vi "MD420_ACT_TargetValue.vi"() -> ()   [LabVIEW 2022 SP3, in "MD420.lvclass"]
uses:
  MD420.lvclass
  MD420.lvclass/MD420.ctl
  SI_modules/SI657/SI657.lvclass
  SI_modules/SI656/SI656.lvclass
  SI_modules/SI101/SI101_AverageReactorCoolantTemperature.lvclass
panel:
  in  "Redundacy Inputs":T1
  out "error IO":errorcluster
  in  "error in (no error)":errorcluster
  out "SI101_AverageReactorCoolantTemperature.lvclass out":refnum<class "SI101_AverageReactorCoolantTemperature.lvclass">
  out "SI657.lvclass out":refnum<class "SI657.lvclass">
  out "SI656 out":refnum<class "SI656.lvclass">
  in  "Loop Meas":T2
  in  "From Turbine SI656":T3
  in  "From Turbine SI657":T4
  in  "SI101_AverageReactorCoolantTemperature.lvclass":refnum<class "SI101_AverageReactorCoolantTemperature.lvclass">
  in  "SI656.lvclass":refnum<class "SI656.lvclass">
  in  "SI657.lvclass":refnum<class "SI657.lvclass">
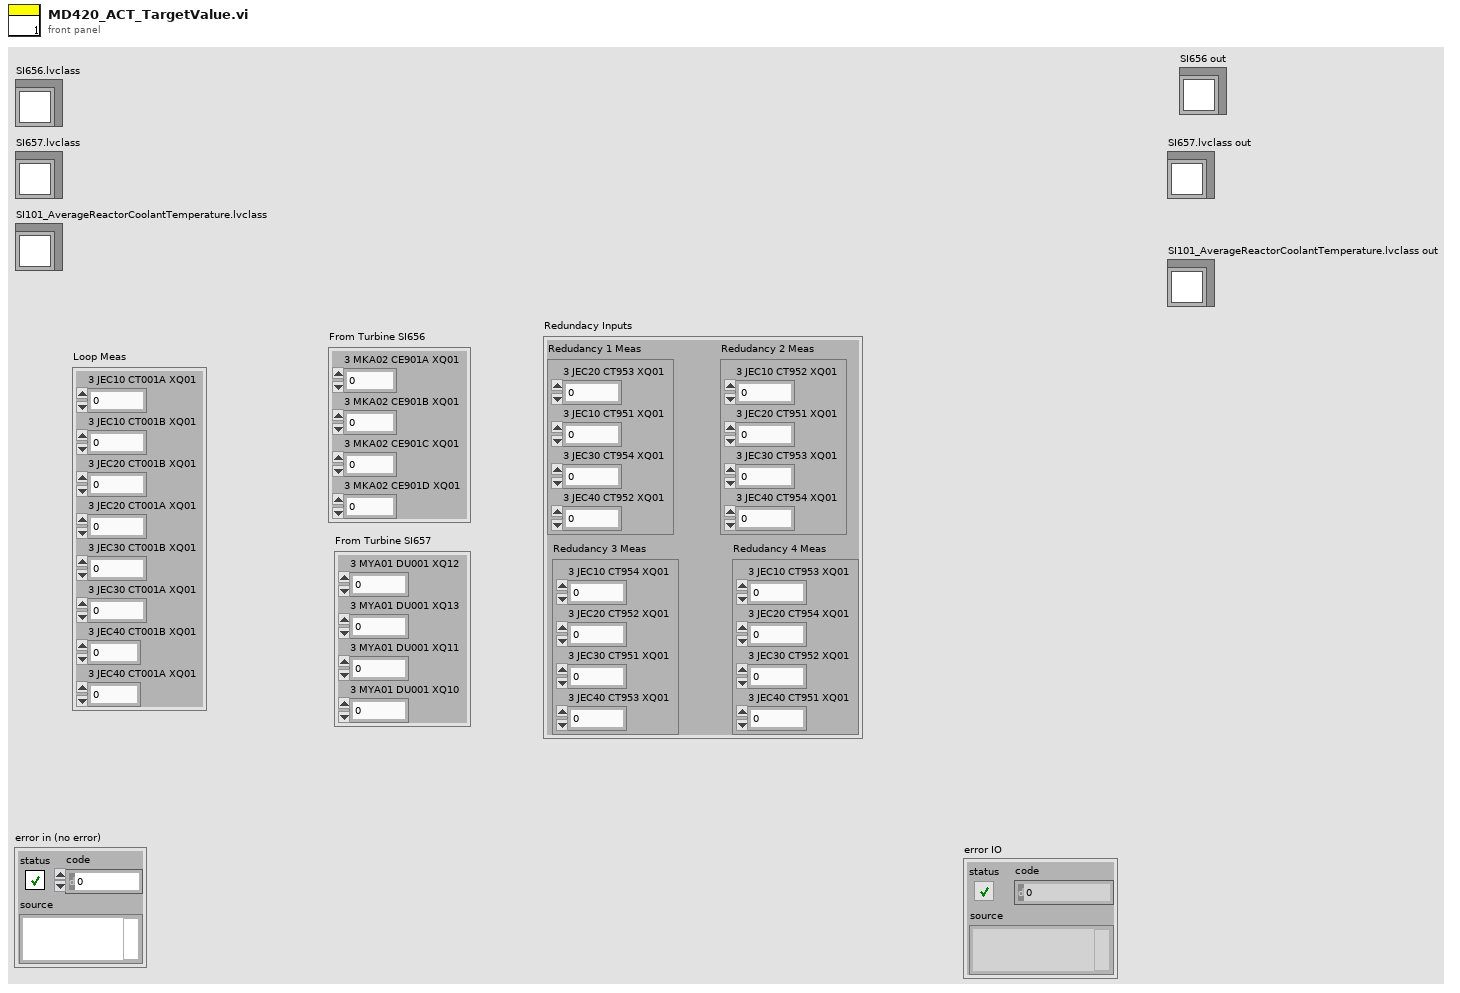
[diagram p1: front panel]
types:
  T1 = cluster{"Redudancy 1 Meas":cluster{"3 JEC20 CT953 XQ01":dbl, "3 JEC10 CT951 XQ01":dbl, "3 JEC30 CT954 XQ01":dbl, "3 JEC40 CT952 XQ01":dbl}, "Redudancy 2 Meas":cluster{"3 JEC10 CT952 XQ01":dbl, "3 JEC20 CT951 XQ01":dbl, "3 JEC30 CT953 XQ01":dbl, "3 JEC40 CT954 XQ01":dbl}, "Redudancy 3 Meas":cluster{"3 JEC10 CT954 XQ01":dbl, "3 JEC20 CT952 XQ01":dbl, "3 JEC30 CT951 XQ01":dbl, "3 JEC40 CT953 XQ01":dbl}, "Redudancy 4 Meas":cluster{"3 JEC10 CT953 XQ01":dbl, "3 JEC20 CT954 XQ01":dbl, "3 JEC30 CT952 XQ01":dbl, "3 JEC40 CT951 XQ01":dbl}}
  T2 = cluster{"3 JEC10 CT001A XQ01":dbl, "3 JEC10 CT001B XQ01":dbl, "3 JEC20 CT001B XQ01":dbl, "3 JEC20 CT001A XQ01":dbl, "3 JEC30 CT001B XQ01":dbl, "3 JEC30 CT001A XQ01":dbl, "3 JEC40 CT001B XQ01":dbl, "3 JEC40 CT001A XQ01":dbl}
  T3 = cluster{"3 MKA02 CE901A XQ01":dbl, "3 MKA02 CE901B XQ01":dbl, "3 MKA02 CE901C XQ01":dbl, "3 MKA02 CE901D XQ01":dbl}
  T4 = cluster{"3 MYA01 DU001 XQ12":dbl, "3 MYA01 DU001 XQ13":dbl, "3 MYA01 DU001 XQ11":dbl, "3 MYA01 DU001 XQ10":dbl}
  T5 = cluster{"3 JEC20 CT953 XQ01":dbl, "3 JEC10 CT951 XQ01":dbl, "3 JEC30 CT954 XQ01":dbl, "3 JEC40 CT952 XQ01":dbl}
  T6 = cluster{"3 JEC10 CT952 XQ01":dbl, "3 JEC20 CT951 XQ01":dbl, "3 JEC30 CT953 XQ01":dbl, "3 JEC40 CT954 XQ01":dbl}
  T7 = cluster{"3 JEC10 CT954 XQ01":dbl, "3 JEC20 CT952 XQ01":dbl, "3 JEC30 CT951 XQ01":dbl, "3 JEC40 CT953 XQ01":dbl}
  T8 = cluster{"3 JEC10 CT953 XQ01":dbl, "3 JEC20 CT954 XQ01":dbl, "3 JEC30 CT952 XQ01":dbl, "3 JEC40 CT951 XQ01":dbl}
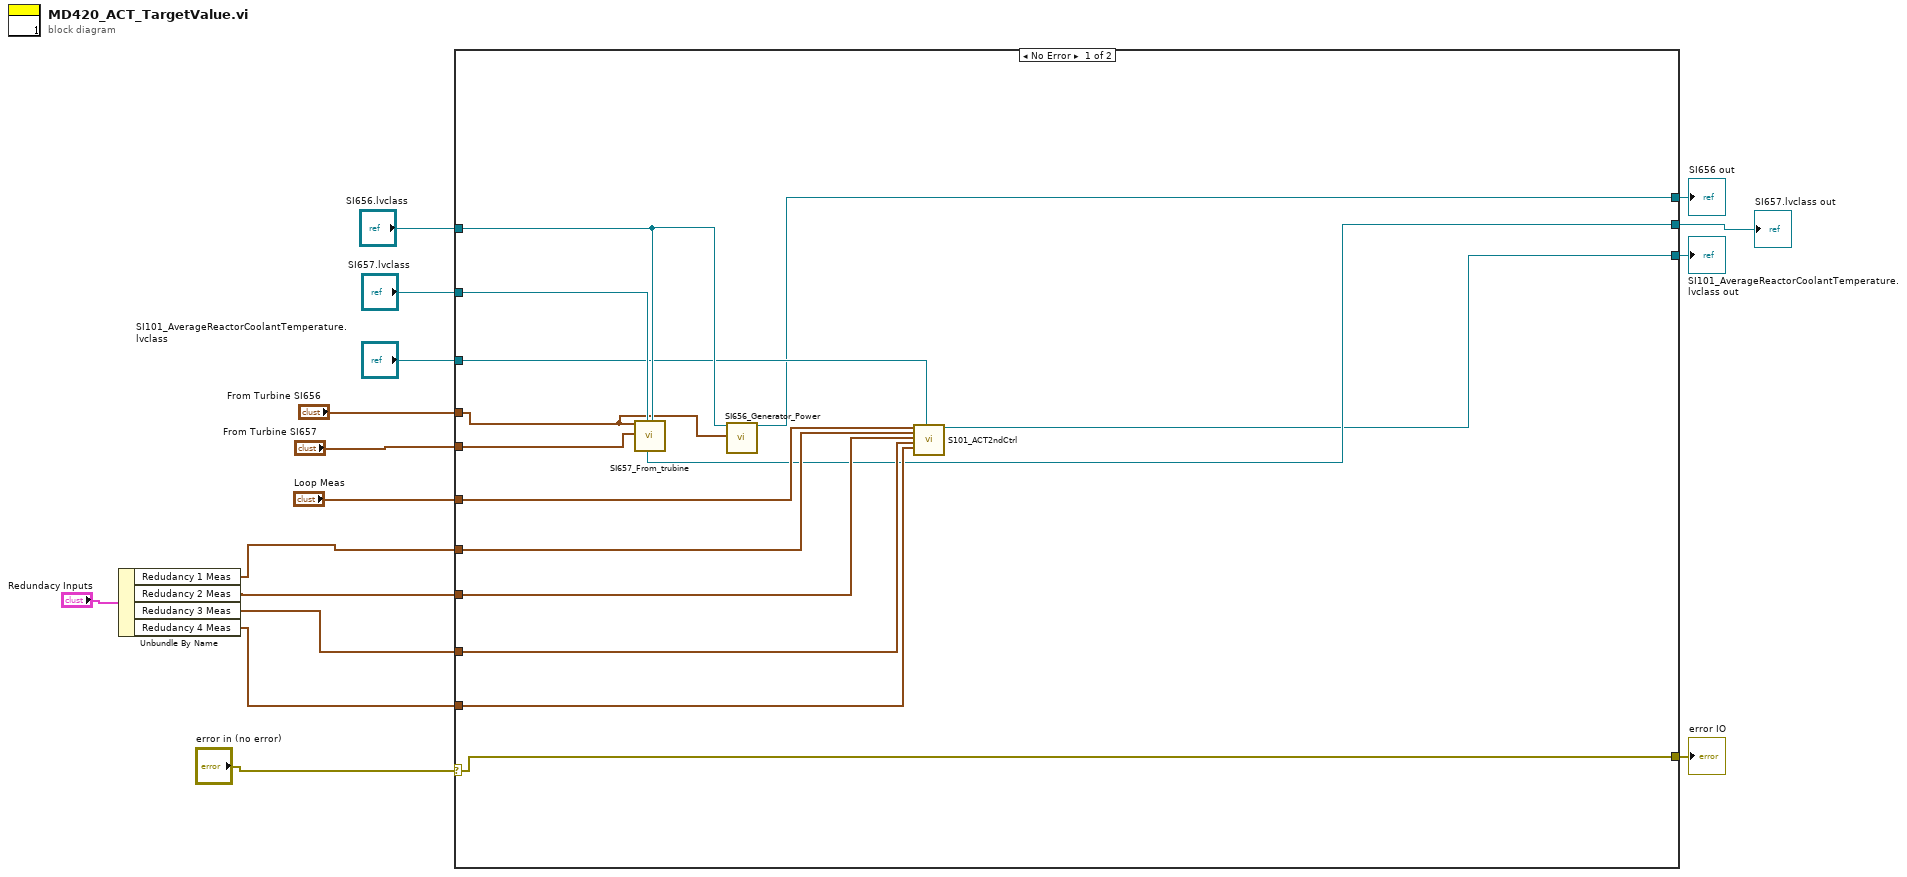
[diagram p0: block diagram]
diagram:
  n1 = Unbundle By Name("Redundacy Inputs") -> ("Redudancy 1 Meas"=w4:T5, "Redudancy 2 Meas"=w3:T6, "Redudancy 3 Meas"=w2:T7, "Redudancy 4 Meas"=w1:T8)
  n2 = case shown="No Error" "error in (no error)" {
    selector: "error in (no error)" -> [w17 w31]
    tunnel: "SI657.lvclass" -> [w30 _]
    tunnel: "SI656.lvclass" -> [w28 _]
    tunnel: "SI101_AverageReactorCoolantTemperature.lvclass" -> [w26 _]
    tunnel: "From Turbine SI656" -> [w27 _]
    tunnel: "From Turbine SI657" -> [w29 _]
    tunnel: "Loop Meas" -> [w25 _]
    tunnel: w4 -> [w24 _]
    tunnel: w3 -> [w23 _]
    tunnel: w2 -> [w22 _]
    tunnel: w1 -> [w21 _]
    tunnel: [w20 _] -> w9
    tunnel: [w19 _] -> w10
    tunnel: [w18 _] -> w8
    tunnel: [w17 w31] -> w6
    frame No Error {
      n3 = call "SI657_From_trubine.vi"("From Turbine SI656"=w27, "From Turbine SI657"=w29, "SI657.lvclass"=w30, "SI656.lvclass"=w28) -> ("SI657.lvclass out"=w20:refnum<class "SI657.lvclass">)  [unwired: 8 in, 7 out]
      n4 = call "SI656_Generator_Power.vi"("SI656 in"=w28, "From Turbine"=w27) -> ("SI656 out"=w19:refnum<class "SI656.lvclass">)  [unwired: 14 in, 3 out]
      n5 = call "S101_ACT2ndCtrl.vi"("Loop Meas"=w25, "Redudancy 1 Meas"=w24, "Redudancy 2 Meas"=w23, "Redudancy 3 Meas"=w22, "Redudancy 4 Meas"=w21, "SI101_AverageReactorCoolantTemperature.lvclass"=w26) -> ("SI101_AverageReactorCoolantTemperature.lvclass out"=w18:refnum<class "SI101_AverageReactorCoolantTemperature.lvclass">)  [unwired: 10 in, 3 out]
    }
    frame Error {
    }
  }
  "SI656 out" <- w10
  "SI657.lvclass out" <- w9
  "SI101_AverageReactorCoolantTemperature.lvclass out" <- w8
  "error IO" <- w6
